vi "Perform ac dual channel measurement.vi"(8 "error in":errorcluster, 10 "I2S waveforms":waveform(dbl)[](array[waveform]), 11 "measurement configuration":T2={"Band start"=20.0, "Band stop"=20000.0, "Weighting Filter"=enum."Linear", "Full scale range"=2.825, "Left channel name"="", "Right channel name"="", "Left channel analog source resource name"="", "Right channel analog source resource name"="", "Frequency"=1000.0, "Amplitude"=-1.0, "Protocol capture resource name"="", "Data line"=0, "Left acquisition channel"=0, "Right acquisition channel"=0, "Sample rate"=44100.0, "Measurement Duration"=0.1, "Frame sync edge for Channel 0"=enum."Falling", "Channel count per frame"=2, "Channel length"=32, "Bit depth"=24, "Channel 0 offset"=1, "Endianness"=enum."MSB First", "Data Justification"=enum."Left Justified", "Frame length"=64, "Frame sync pulse width"=32, "Bit clock edge  sync"=enum."Falling"} {"Frame length" format="%#_6ps"}) -> (0 "error out":errorcluster, 3 "measurement results":T1)   [LabVIEW 2021, in "AC Dual Channel_Audio ADC.lvlib"]
uses:
  AC Dual Channel_Audio ADC.lvlib
  Measurement Configuration.ctl
  Measurement Results.ctl
  <vilib>/addons/_NISVFA/_Shared subVIs/Controls/svc_Window.ctl
  <vilib>/addons/_NISVFA/_Shared subVIs/Common/SVL Set dB Reference (N Ch - 1 Ref).vi
  <vilib>/addons/Sound and Vibration/svt_Level/SVL AC & DC Level (Time) (N Ch).vi
  <vilib>/addons/Sound and Vibration/svt_Single Tone Measurements/SVT Spurious Free Dynamic Range (Frequency) (1 Ch).vi
  <vilib>/addons/_NISVFA/_Spectrum Processing/SVFA Unit Conversion (Complex) (1 Ch).vi
  <vilib>/addons/_NISVFA/_Shared subVIs/Common/SVL Set dB Reference (1 Ch).vi
  <vilib>/addons/Sound and Vibration/svt_Level/SVL AC & DC Level (Time) (1 Ch).vi
  <vilib>/addons/_NISVFA/_Spectrum Processing/SVFA Get Spectrum Subset.vi
  <vilib>/addons/_NISVFA/_Spectrum Processing/SVFA Get Spectrum Subset (Complex) (1 Ch).vi
  <vilib>/addons/_NISVFA/_Shared subVIs/Common/svc_Window Parameters.vi
  <vilib>/addons/_NISVFA/_Shared subVIs/Common/svc_Extract Single Tone Information (complex).vi
  <vilib>/addons/_NISVFA/_Shared subVIs/Common/svc_Check Frequency Range in Spectrum.vi
  <vilib>/addons/_NISVFA/_Spectrum Processing/SVFA Spectrum Peak Search.vi
  <vilib>/addons/_NISVFA/_Spectrum Processing/SVFA Spectrum Peak Search (1 Ch).vi
  <vilib>/addons/_NISVFA/_Shared subVIs/Common/svc_Spectrum Units.vi
  <vilib>/addons/_NISVFA/_Shared subVIs/Common/svc_Log View for Spectrum (1Ch).vi
  <vilib>/addons/_NISVFA/_Spectrum Processing/SVFA Unit Conversion (1 Ch).vi
  <vilib>/addons/_NISVFA/_Shared subVIs/Common/svc_Complex Datatype Defaults.vi
  <vilib>/addons/_NISVFA/_Shared subVIs/Common/svc_Build Unit Label for Frequency Range.vi
  <vilib>/addons/_NISVFA/_Shared subVIs/Common/SVL Set dB Reference (variant).vi
  <vilib>/addons/_NISVFA/_Shared subVIs/Common/svc_Get SV Channel Info.vi
  <vilib>/Analysis/baseanly.llb/Mean.vi
  <vilib>/Analysis/baseanly.llb/Mean (DBL).vi
  <vilib>/addons/_NISVFA/_Shared subVIs/Windowing/svfa_Scaled Time Domain Window (Array).vi
  <vilib>/addons/_NISVFA/_Spectrum Processing/SVFA Get Tone Amplitude and Phase (1 Ch).vi
  <vilib>/addons/_NISVFA/_Spectrum Processing/subVIs/svfa_Compute Complex Spectrum for Export.vi
  <vilib>/addons/_NISVFA/_Shared subVIs/Common/svc_Check Frequency Range in Bandwidth.vi
  <vilib>/addons/_NISVFA/_Shared subVIs/Common/svc_Convert Start and Stop to Start Index and Length.vi
  <vilib>/addons/_NISVFA/_Spectrum Processing/subVIs/svfa_Spectrum Peak Search.vi
  <vilib>/addons/_NISVFA/_Shared subVIs/Common/svc_Format Value (DBL).vi
  <vilib>/addons/_NISVFA/_Shared subVIs/Common/svc_Get Weighting Enum and Labels.vi
  <vilib>/addons/_NISVFA/_Shared subVIs/Common/svc_Engineering Units to Unit Label.vi
  <vilib>/addons/_NISVFA/_Shared subVIs/Common/svc_Surround NonAlpha String with Parentheses.vi
  <vilib>/dlg_ctls.llb/Space Constant.vi
  <vilib>/addons/_NISVFA/_Shared subVIs/Common/svc_Unwrap Phase.vi
  <vilib>/addons/_NISVFA/_Shared subVIs/Common/svc_Convert Spectrum Array to dB.vi
  <vilib>/addons/_NISVFA/_Spectrum Processing/subVIs/svfa_Conversion Utility (spectrum info).vi
  <vilib>/addons/_NISVFA/_Shared subVIs/Common/svc_Unit Label to Engineering Units.vi
  <vilib>/addons/_NISVFA/_Spectrum Processing/subVIs/svfa_Spectrum Info Window to windowTd Type Def.vi
  <vilib>/Analysis/4window.llb/Force Window.vi
  <vilib>/Analysis/4window.llb/Force Window (DBL).vi
  <vilib>/Analysis/4window.llb/Exponential Window.vi
  <vilib>/Analysis/4window.llb/Exponential Window (DBL).vi
  <vilib>/addons/_NISVFA/_Spectrum Processing/subVIs/svfa_Window Frequency Response.vi
  <vilib>/addons/_NISVFA/_Spectrum Processing/subVIs/svfa_Window Frequency Response (double array).vi
  <vilib>/Analysis/baseanly.llb/Dot Product.vi
  <vilib>/Analysis/baseanly.llb/Complex Dot Product.vi
  <vilib>/addons/_NISVFA/_Spectrum Processing/subVIs/svfa_Peak Rough Search Indices.vi
  <vilib>/addons/_NISVFA/_Shared subVIs/Common/svc_Unit Label Lexical Class.vi
  <vilib>/addons/_NISVFA/_Spectrum Processing/subVIs/svfa_Peak to RMS to Peak2Peak.vi
  <vilib>/addons/_NISVFA/_Spectrum Processing/subVIs/svfa_Mag to Mag2.vi
  <vilib>/addons/_NISVFA/_Spectrum Processing/subVIs/svfa_Linear to dB.vi
  <vilib>/addons/_NISVFA/_Spectrum Processing/subVIs/svfa_dBrefA to dBrefB.vi
  <vilib>/addons/_NISVFA/_Spectrum Processing/subVIs/svfa_Spectrum to Spectral Density.vi
  <vilib>/addons/_NISVFA/_Spectrum Processing/subVIs/svfa_Rect Window Frequency Response.vi
  <vilib>/addons/_NISVFA/_Spectrum Processing/subVIs/svfa_Cosine Window Coefficients.vi
  <vilib>/addons/Sound and Vibration/svt_Weighting/SVT Weighting Filter (N Ch).vi
  <vilib>/addons/_NISVFA/_Shared subVIs/Common/svc_Caller VI Returned in Error Source.vi
  <vilib>/addons/_NISVFA/_Shared subVIs/Common/svc_Get Window Info.vi
  <vilib>/Analysis/0measdsp.llb/Scaled Time Domain Window.vi
  <vilib>/Analysis/0measdsp.llb/Scaled Time Domain Window (DBL).vi
  <vilib>/Utility/error.llb/Error Cluster From Error Code.vi
  <vilib>/Analysis/baseanly.llb/Std Deviation and Variance.vi
  <vilib>/addons/Sound and Vibration/svt_Single Tone Measurements/SVT Gain (Time) (1 Ch).vi
  <vilib>/addons/Sound and Vibration/svt_Distortion/SVT SNR without Harmonics (Frequency) (1 Ch).vi
  <vilib>/addons/Sound and Vibration/svt_Single Tone Measurements/SVT Dynamic Range (Frequency) (1 Ch).vi
  <vilib>/addons/Sound and Vibration/svt_Distortion/subVIs/sv_Check Data Valid (Audio) (1 Ch).vi
  <vilib>/addons/_NISVFA/_Shared subVIs/Common/svc_Convert Frequency to Frequency String.vi
  <vilib>/Analysis/4window.llb/window parameters.vi
  <vilib>/Analysis/4window.llb/Window Properties.vi
  <vilib>/Analysis/4window.llb/Window Properties by Name.vi
  <vilib>/addons/_NISVFA/_Spectrum Processing/subVIs/svfa_Spectrum Peak Tone Search and Estimation (complex).vi
  <vilib>/measure/masignal.llb/Tones and Noise Waveform.vi
  <vilib>/addons/_NISVFA/_Shared subVIs/Common/svc_FFT with Window.vi
  <vilib>/Analysis/1siggen.llb/Square Wave.vi
  <vilib>/addons/_NISVFA/_Spectrum Processing/subVIs/svfa_Three Finger Peak Search.vi
  <vilib>/addons/Sound and Vibration/svt_Distortion/subVIs/sv_Peak View Amplitude (1 Ch).vi
  <vilib>/addons/Sound and Vibration/svt_Weighting/SoundVib_ABCWeighting.lvlib
  <vilib>/addons/Sound and Vibration/svt_Single Tone Measurements/SoundVib_SingleTone.lvlib
  <vilib>/addons/Sound and Vibration/svt_Distortion/SoundVib_Distortion.lvlib
  shared/Audio ADC Shared.lvlib
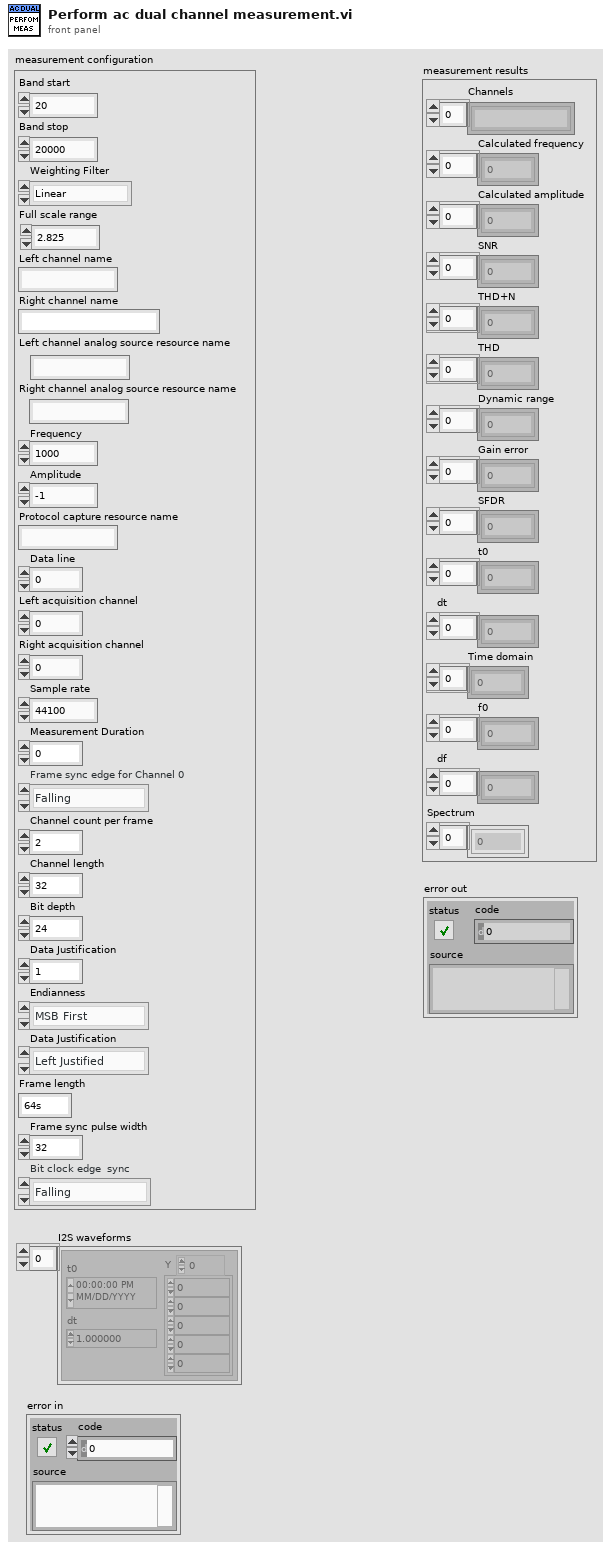
[diagram p1: front panel]
types:
  T1 = typedef "AC Dual Channel_Audio ADC.lvlib/Measurement Results.ctl" = cluster{"Channels":string[], "Calculated frequency":dbl[], "Calculated amplitude":dbl[], "SNR":dbl[], "THD+N":dbl[], "THD":dbl[], "Dynamic range":dbl[], "Gain error":dbl[], "SFDR":dbl[], "t0":dbl[], "dt":dbl[], "Time domain":dbl[], "f0":dbl[], "df":dbl[], "Spectrum":dbl[]}
  T2 = typedef "AC Dual Channel_Audio ADC.lvlib/Measurement Configuration.ctl" = cluster{"Band start":dbl, "Band stop":dbl, "Weighting Filter":enum32{"Linear", "A-weighting", "B-weighting", "C-weighting"}, "Full scale range":dbl, "Left channel name":string, "Right channel name":string, "Left channel analog source resource name":string, "Right channel analog source resource name":string, "Frequency":dbl, "Amplitude":dbl, "Protocol capture resource name":string, "Data line":i32, "Left acquisition channel":i32, "Right acquisition channel":i32, "Sample rate":dbl, "Measurement Duration":dbl, "Frame sync edge for Channel 0":enum32{"Rising", "Falling"}, "Channel count per frame":u32, "Channel length":u32, "Bit depth":u32, "Channel 0 offset":u32, "Endianness":enum32{"MSB First", "LSB First"}, "Data Justification":enum32{"Left Justified", "Right Justified"}, "Frame length":u32, "Frame sync pulse width":u32, "Bit clock edge  sync":enum32{"Rising", "Falling"}}
  T3 = cluster{"start frequency":dbl, "stop frequency":dbl}
  T4 = typedef "svc_Window.ctl" = u32
  T5 = enum32{"Linear", "A-weighting", "B-weighting", "C-weighting"}
  T6 = enum16{"no change", "spectrum", "spectral density"}
  T7 = cluster{"linear/dB":enum16{"no change", "linear", "dB"}, "dB reference (0: no change)":dbl, "power/magnitude":enum16{"no change", "power", "magnitude"}, "view":enum16{"no change", "rms", "peak", "peak-peak"}}
  T8 = cluster{"gain units":enum16{"dB", "linear ratio"}, "detected fundamental amplitude units":enum16{"EU rms", "EU peak", "EU peak-peak"}}
  T9 = cluster{"SNR units":enum16{"dB", "linear ratio", "%"}, "detected fundamental amplitude units":enum16{"EU rms", "EU peak", "EU peak-peak"}}
  T10 = typedef "svc_Spectrum Info.ctl" = cluster{"channel name":string, "description":string, "x-axis units":T11, "spectral info":cluster{"spectrum type":T12, "linear/dB":enum16{"linear", "dB"}, "window":u16, "window size":i32, "FFT size":i32}, "engineering units":T13, "custom label":string, "dB reference [EU]":dbl, "peak units":enum16{"rms", "peak", "peak-peak"}, "weighting filter":T14, "spectral density?":bool, "unit label":string, "spectrum skewed?":bool, "complimentary spectrum units":T15}
  T11 = typedef "svc_X-Axis Units.ctl" = u16
  T12 = typedef "svc_Spectrum Type.ctl" = enum16{"FFT Spectrum [complex]", "Amplitude [Magnitude]", "Power [Magnitude^2]", "Cross Spectrum [complex]", "Frequency Response [Complex]"}
  T13 = typedef "svc_Engineering Units Text Ring.ctl" = u16
  T14 = typedef "svc_Weighting Filter Text Ring.ctl" = u16
  T15 = typedef "svc_Complimentary Spectrum Units.ctl" = enum16{"none", "radians", "degrees", "cycles", "imaginary"}
  T16 = cluster{"complex spectrum response":cluster{"f0":dbl, "df":dbl, "complex spectrum":cdb[]}, "spectrum info":T10}
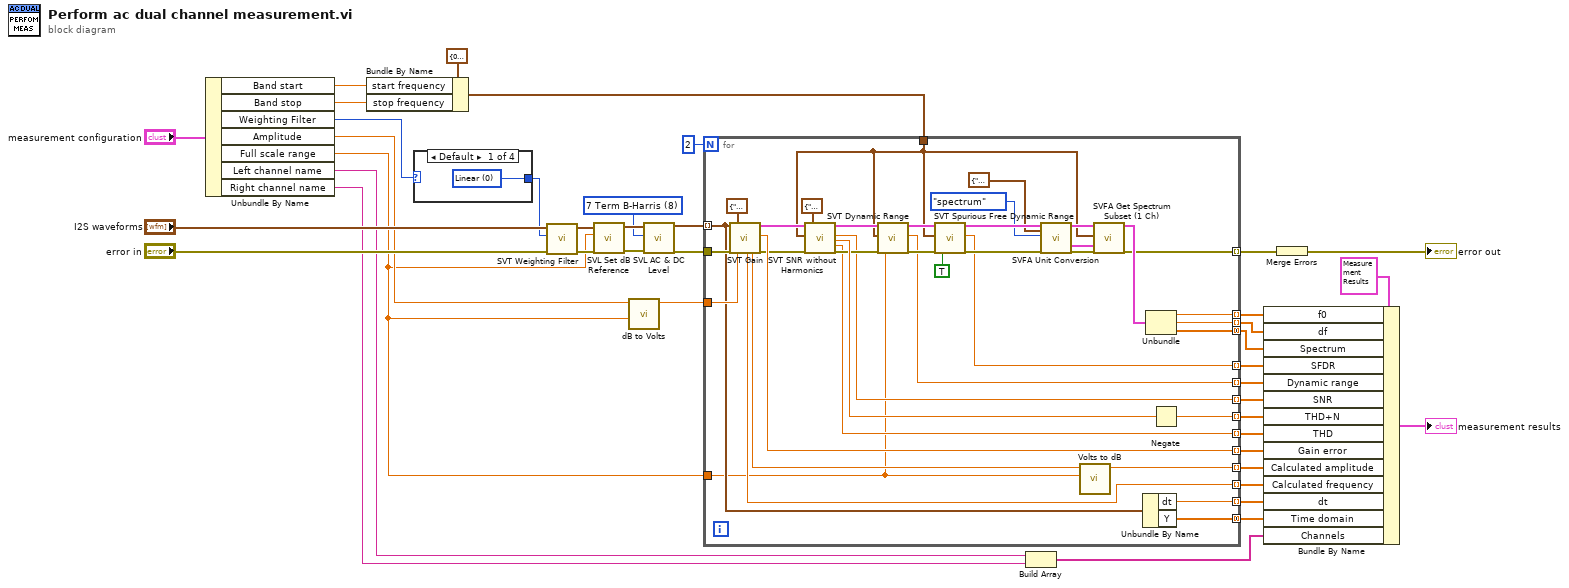
[diagram p0: block diagram]
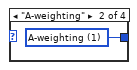
[diagram p2: hidden frame]
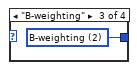
[diagram p3: hidden frame]
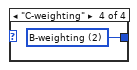
[diagram p4: hidden frame]
diagram:
  w28 = T4 8 items=["None"=0, "Hanning"=1, "Hamming"=2, "Blackman-Harris"=3, "Exact Blackman"=4, "Blackman"=5, "Flat Top"=6, "4 Term B-Harris "=7, "7 Term B-Harris"=8, "Low Sidelobe"=9, "Force"=64, "Exponential"=65, "Blackman Nuttall"=11, "Triangle"=30, "Bartlett-Hanning"=31, "Bohman"=32, "Parzen"=33, "Welch"=34, "Kaiser"=60, "Dolph-Chebyshev"=61, "Gaussian"=62] ("window")
  n1 = Unbundle By Name("measurement configuration") -> ("Band start"=w36:dbl, "Band stop"=w37:dbl, "Weighting Filter"=w21:T5, "Amplitude"=w7:dbl, "Full scale range"=w5:dbl, "Left channel name"=w4:string, "Right channel name"=w3:string)
  n2 = Bundle By Name(cluster=T3 {"start frequency"=0.0, "stop frequency"=0.0} ("frequency range"), "start frequency"=w36, "stop frequency"=w37) -> (w23:T3)
  n3 = case shown="Default" w21 {
    tunnel: [w41 w42 w43 w44] -> w20
    frame Default {
      w41 = u16 0 items=["Linear", "A-weighting", "B-weighting", "C-weighting"] ("weighting")
    }
    frame "A-weighting" {
      w42 = u16 1 items=["Linear", "A-weighting", "B-weighting", "C-weighting"] ("weighting")
    }
    frame "B-weighting" {
      w43 = u16 2 items=["Linear", "A-weighting", "B-weighting", "C-weighting"] ("weighting")
    }
    frame "C-weighting" {
      w44 = u16 2 items=["Linear", "A-weighting", "B-weighting", "C-weighting"] ("weighting")
    }
  }
  n4 = call-poly <vilib>:"SVT Weighting Filter.vi"("error in (no error)"="error in", "weighting"=w20, "scaled signals [EU]"="I2S waveforms") -> ("error out"=w33:errorcluster, "weighted signals [EU]"=w32:waveform(dbl)[])  [unwired: 6 in]
  n5 = call-poly <vilib>:"SVL Set dB Reference.vi"("error in (no error)"=w33, "dB reference [EU]"=w5, "scaled signals in [EU]"=w32) -> ("error out"=w29:errorcluster, "scaled signals out [EU]"=w30:waveform(dbl)[])  [unwired: 7 in]
  n6 = call "dB to Volts.vi"("Full scale range"=w5, "Voltage(dB)"=w7) -> ("Voltage(volts)"=w6:dbl)  [unwired: 9 in]
  n7 = call-poly <vilib>:"SVL AC & DC Level.vi"("scaled signals in [EU]"=w30, "window"=w28, "error in (no error)"=w29) -> ("AC signals [EU]"=w12:waveform(dbl)[], "error out"=w31:errorcluster)  [unwired: 11 in, 4 out]
  n8 = for {
    N: 2 -> [_]
    tunnel: [w82] -> w40 mode=concatenating
    tunnel: [w81] -> w39 mode=indexing
    tunnel: [w80] -> w38 mode=indexing
    tunnel: [w64] -> w26 mode=indexing
    tunnel: [w63] -> w25 mode=indexing
    tunnel: [w62] -> w24 mode=concatenating
    tunnel: w6 -> [w61]
    tunnel: w23 -> [w59]
    tunnel: w5 -> [w46]
    tunnel: [w54] -> w19 mode=indexing
    tunnel: [w53] -> w18 mode=indexing
    tunnel: [w52] -> w17 mode=indexing
    tunnel: [w51] -> w16 mode=indexing
    tunnel: [w50] -> w15 mode=indexing
    tunnel: [w45] -> w14 mode=indexing
    tunnel: [w49] -> w13 mode=indexing
    tunnel: w12 -> [w48] mode=indexing
    tunnel: w31 -> [w76]
    tunnel: [w57] -> w22 mode=indexing
    n9 = call-poly <vilib>:"SVT Gain.vi"("scaled signal [EU]"=w48, "error in (no error)"=w76, "desired units"=T8 {"gain units"=enum."dB", "detected fundamental amplitude units"=enum."EU peak"}, "amplitude [EU peak]"=w61) -> ("detected fundamental\nfrequency [Hz]"=w49:dbl, "detected fundamental\namplitude"=w47:dbl, "complex spectrum"=w69:T16, "gain"=w80:dbl, "error out"=w70:errorcluster)  [unwired: 10 in, 1 out]
    n10 = call-poly <vilib>:"SVT SNR without Harmonics.vi"("complex spectrum"=w69, "frequency range"=w59, "error in (no error)"=w70, "desired units"=T9 {"SNR units"=enum."dB", "detected fundamental amplitude units"=enum."EU rms"}) -> ("complex spectrum"=w72:T16, "SNR (without harmonics)"=w52:dbl, "SINAD"=w73:dbl, "THD"=w50:dbl, "error out"=w71:errorcluster)  [unwired: 8 in, 3 out]
    n11 = call-poly <vilib>:"SVT Dynamic Range.vi"("complex spectrum"=w72, "frequency range"=w59, "error in (no error)"=w71, "full scale amplitude [EU peak]"=w46) -> ("dup complex spectrum"=w77:T16, "dynamic range"=w53:dbl, "error out"=w78:errorcluster)  [unwired: 10 in, 3 out]
    n12 = call-poly <vilib>:"SVT Spurious Free Dynamic Range.vi"("complex spectrum"=w77, "frequency range"=w59, "error in (no error)"=w78, "exclude harmonics"=TRUE) -> ("complex spectrum"=w67:T16, "spurious free dynamic range"=w54:dbl, "error out"=w68:errorcluster)  [unwired: 8 in, 5 out]
    n13 = call-poly <vilib>:"SVFA Unit Conversion.vi"("complex spectrum"=w67, "desired scaling"=T7 {"linear/dB"=enum."dB", "dB reference (0: no change)"=0.0, "power/magnitude"=enum."magnitude", "view"=enum."peak-peak"}, "spectral density desired"=T6."spectrum", "error in (no error)"=w68) -> ("converted spectrum"=w60:cluster{"x0":dbl, "dx":dbl, "magnitude":dbl[]}, "spectrum info out"=w56:T10, "error out"=w55:errorcluster)  [unwired: 10 in, 3 out]
    n14 = call "Volts to dB.vi"("Full scale range"=w46, "Voltage(V)"=w47) -> ("Voltage(dB)"=w45:dbl)  [unwired: 9 in]
    n15 = call <vilib>:"SVFA Get Spectrum Subset (1 Ch).vi"("spectrum"=w60, "range"=w59, "spectrum info"=w56, "error in (no error)"=w55) -> ("spectrum subset"=w58:cluster{"x0":dbl, "dx":dbl, "magnitude":dbl[]}, "error out"=w57:errorcluster)  [unwired: 10 in, 4 out]
    n16 = Unbundle By Name ("Get Waveform Components")(w48) -> ("dt"=w81:dbl, "Y"=w82:dbl[])
    n17 = Unbundle(w58) -> ("x0"=w64:dbl, "dx"=w63:dbl, "magnitude"=w62:dbl[])
    n18 = Negate(x=w73) -> (-x=w51:dbl)
  }
  n19 = Build Array(w4, w3) -> (w2:string[])
  n20 = Bundle By Name(cluster=T1 {"Channels"=[], "Calculated frequency"=[], "Calculated amplitude"=[], "SNR"=[], "THD+N"=[], "THD"=[], "Dynamic range"=[], "Gain error"=[], "SFDR"=[], "t0"=[], "dt"=[], "Time domain"=[], "f0"=[], "df"=[], "Spectrum"=[]} ("measurement results"), "f0"=w26, "df"=w25, "Spectrum"=w24, "SFDR"=w19, "Dynamic range"=w18, "SNR"=w17, "THD+N"=w16, "THD"=w15, "Gain error"=w38, "Calculated amplitude"=w14, "Calculated frequency"=w13, "dt"=w39, "Time domain"=w40, "Channels"=w2) -> (→"measurement results":T1)
  n21 = Merge Errors(w22) -> (→"error out":errorcluster)
